vi "feet to encoder ticsk.vi"(11 "Distance in feet wanted":dbl) -> (3 "Encoder Ticks":dbl)   [LabVIEW 2017]
panel:
  # "Dosen't do anything right now"
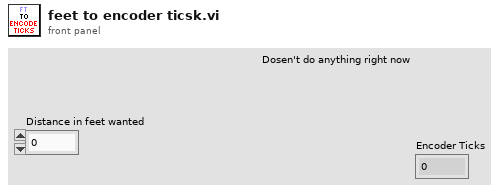
[diagram p1: front panel]
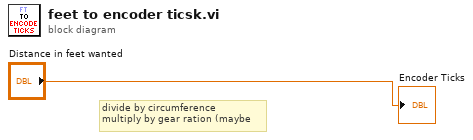
[diagram p0: block diagram]
diagram:
  # "divide by circumference\nmultiply by gear ration (maybe"
  "Encoder Ticks" <- "Distance in feet wanted"
